vi "Keithley_VISA_Write_Only.vi"(8 "error in (no error)":errorcluster, 9 "milliseconds to wait":u32, 10 "command":string, 11 "VISA resource name":refnum<visa-resource-name>) -> (0 "error out":errorcluster, 3 "VISA resource name out":refnum<visa-resource-name>)   [LabVIEW 2018]
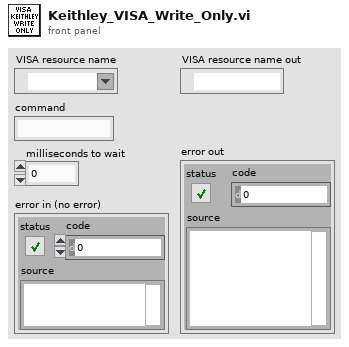
[diagram p1: front panel]
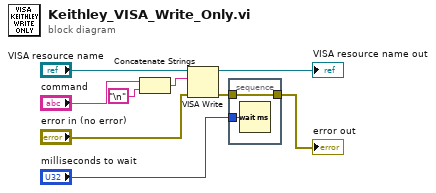
[diagram p0: block diagram]
diagram:
  n1 = Concatenate Strings("command", "\n") -> (w8:string)
  n2 = VISA Write(VISA resource name="VISA resource name", write buffer=w8, error in (no error)="error in (no error)") -> (VISA resource name out=→"VISA resource name out":refnum<visa-resource-name>, error out=w7:errorcluster)  [unwired: 1 out]
  n3 = stacked-sequence {
    tunnel: w7 -> [w11]
    tunnel: [w11] -> w1
    tunnel: "milliseconds to wait" -> [w10]
    frame #0 {
      n4 = Wait (ms)(milliseconds to wait=w10) -> ()  [unwired: 1 out]
    }
  }
  "error out" <- w1
